vi "Save.vi"(6 "Force Single Line(T)":bool=TRUE, 7 "Channel Prefix(\"\")":string, 8 "error in (no error)":errorcluster, 9 "Group Prefix (\"\")":string, 10 "TDMS in":refnum<k34>, 11 "Data to Save":refnum<class "Data.lvclass">) -> (0 "error out":errorcluster, 2 "TDMS Out":refnum<k34>)   [LabVIEW 2020, in "TDMS.lvlib"]
doc: "Save 'Data to Save' to 'TDMS in'."
uses:
  TDMS.lvlib
  PPL/HDH.Data.Generic.lvlibp/Data.lvclass
  PPL/HDH.Data.Generic.lvlibp/Generic Data/Generic Array Data/Generic Array Data.lvclass
  PPL/HDH.Data.Generic.lvlibp/Generic Data/Generic Data.lvclass
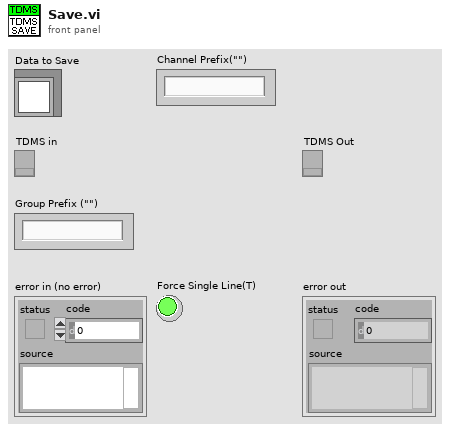
[diagram p1: front panel]
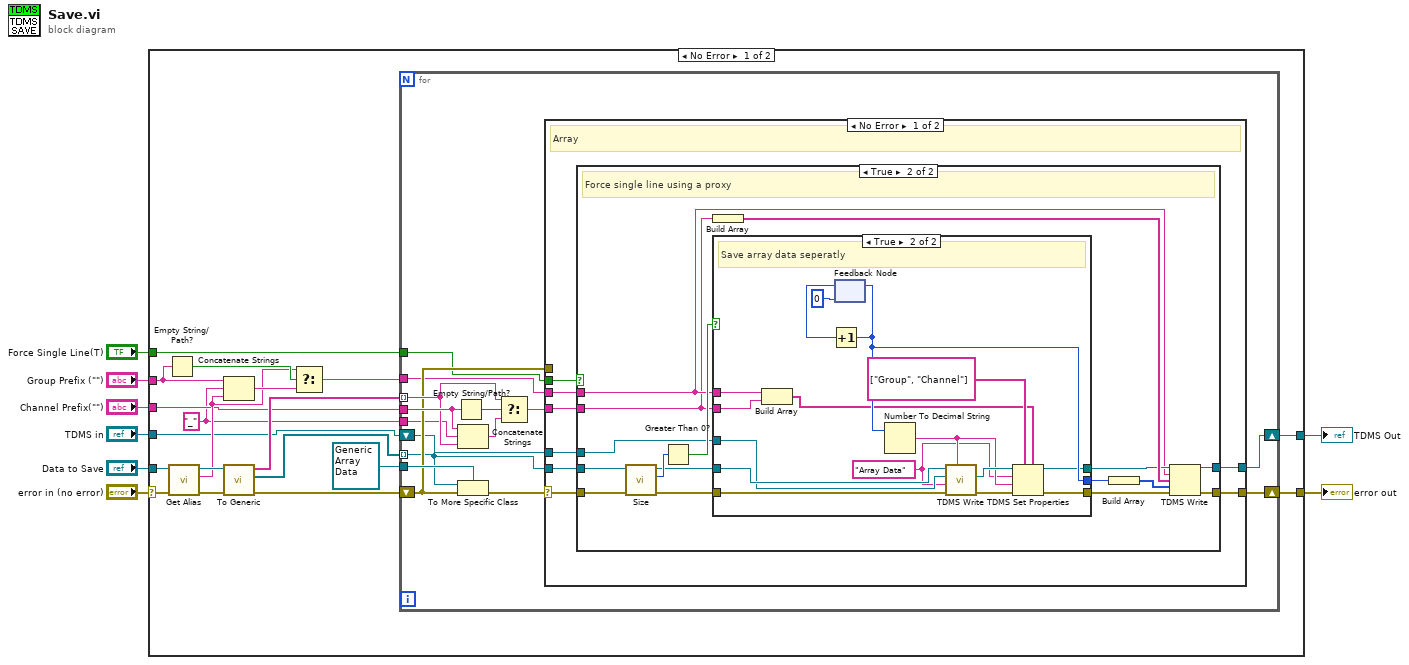
[diagram p0: block diagram]
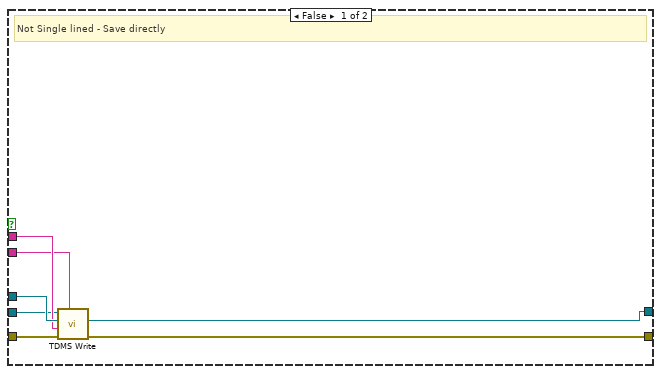
[diagram p2: hidden frame]
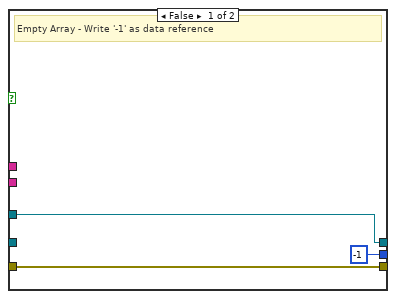
[diagram p3: hidden frame]
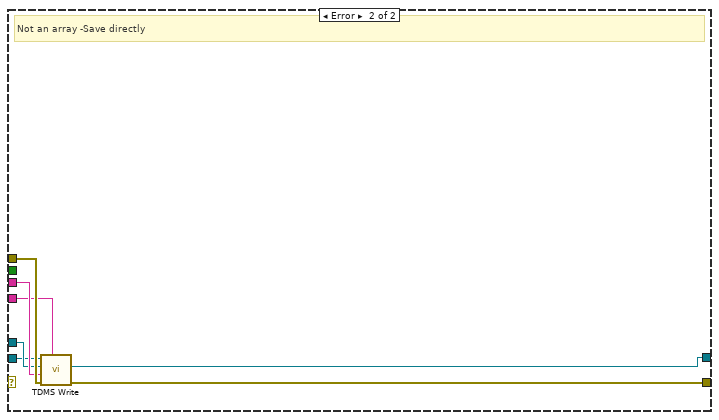
[diagram p4: hidden frame]
diagram:
  n1 = case shown="No Error" "error in (no error)" {
    selector: "error in (no error)" -> [w22 w101]
    tunnel: "Data to Save" -> [w27 _]
    tunnel: [w11 w101] -> w6
    tunnel: [w12 w100] -> w5
    tunnel: "TDMS in" -> [w13 w100]
    tunnel: "Group Prefix (\"\")" -> [w18 _]
    tunnel: "Channel Prefix(\"\")" -> [w14 _]
    tunnel: "Force Single Line(T)" -> [w10 _]
    frame No Error {
      w9 = "_" ("string")
      n2 = Empty String/Path?(string/path=w18) -> (empty?=w19:bool)
      n3 = call-dynamic "Get Alias.vi"("error in (no error)"=w22, "Data in"=w27) -> ("error out"=w21:errorcluster, "Alias"=w16:string, "Data out"=w26:refnum<class "Data.lvclass">)  [unwired: 7 in]
      n4 = Concatenate Strings(w18, w9, w16) -> (w17:string)
      n5 = call-dynamic "To Generic.vi"("error in (no error)"=w21, "Data in"=w26) -> ("error out"=w20:errorcluster, "Generic Data"=w25:refnum<class "Generic Data.lvclass">[], "Data Name"=w24:string[])  [unwired: 7 in]
      n6 = Select(t=w16, s=w19, f=w17) -> (s? t:f=w15:string)
      n7 = for {
        tunnel: w15 -> [w36]
        tunnel: w25 -> [w31] mode=indexing
        tunnel: w24 -> [w38] mode=indexing
        tunnel: refnum<class "Generic Array Data.lvclass"> refnum ("HDH.Data.Generic.lvlibp:Generic Array Data.lvclass") -> [w42]
        shift-right: [w32] -> w11
        shift-left: w20 -> [w37]
        tunnel: w14 -> [w39]
        shift-right: [w33] -> w12
        shift-left: w13 -> [w34]
        tunnel: w10 -> [w29]
        tunnel: w9 -> [w28]
        n8 = Empty String/Path?(string/path=w39) -> (empty?=w40:bool)
        n9 = Concatenate Strings(w39, w28, w38) -> (w41:string)
        n10 = To More Specific Class(target class=w42, reference=w31, error in=w37) -> (error out=w30:errorcluster)  [unwired: 1 out]
        n11 = Select(t=w38, s=w40, f=w41) -> (s? t:f=w35:string)
        n12 = case shown="No Error" w30 {
          selector: w30 -> [w49 _]
          tunnel: w37 -> [_ w99]
          tunnel: w36 -> [w46 w98]
          tunnel: w35 -> [w45 w97]
          tunnel: w34 -> [w48 w96]
          tunnel: [w47 w95] -> w33
          tunnel: [w43 w94] -> w32
          tunnel: w31 -> [w44 w93]
          tunnel: w29 -> [w50 _]
          frame No Error {
            # "Array"
            n13 = case shown="True" w50 {
              tunnel: w49 -> [w57 w70]
              tunnel: w48 -> [w56 w64]
              tunnel: [w55 w63] -> w47
              tunnel: w46 -> [w54 w59]
              tunnel: w45 -> [w53 w58]
              tunnel: w44 -> [w52 w73]
              tunnel: [w51 w62] -> w43
              frame False {
                # "Not Single lined - Save directly"
                n14 = call-dynamic "TDMS Write.vi"("Channel Name"=w53, "error in (no error)"=w57, "Group Name"=w54, "TDMS in"=w56, "Generic Data in"=w52) -> ("error out"=w51:errorcluster, "TDMS Out"=w55:refnum<k34>)  [unwired: 5 in]
              }
              frame True {
                # "Force single line using a proxy"
                n15 = call-dynamic "Size.vi"("error in (no error)"=w70, "Generic Data in"=w73) -> ("error out"=w61:errorcluster, "Size"=w72:i32, "Generic Data out"=w66:refnum<class "Generic Data.lvclass">)  [unwired: 7 in]
                n16 = Greater Than 0?(x=w72) -> (x > 0?=w71:bool)
                n17 = Build Array(w58) -> (w69:string[])
                n18 = case shown="True" w71 {
                  tunnel: [-1 w90] -> w68
                  tunnel: w66 -> [_ w89]
                  tunnel: [w75 w78] -> w65
                  tunnel: w64 -> [w75 w88]
                  tunnel: w61 -> [w74 w87]
                  tunnel: [w74 w77] -> w60
                  tunnel: w59 -> [_ w81]
                  tunnel: w58 -> [_ w80]
                  frame False {
                    # "Empty Array - Write '-1' as data reference"
                  }
                  frame True {
                    w83 = "Array Data" ("Group Name")
                    # "Save array data seperatly"
                    n19 = Build Array(w81, w80) -> (w79:string[])
                    n20 = feedback #1(0) -> (w91:i32)
                    n21 = Increment(x=w91) -> (x+1=w90:i32)
                    n22 = feedback-in #1(w90) -> ()
                    n23 = Number To Decimal String(number=w90) -> (decimal integer string=w84:string)  [unwired: 1 in]
                    n24 = call-dynamic "TDMS Write.vi"("Channel Name"=w84, "error in (no error)"=w87, "Group Name"=w83, "TDMS in"=w88, "Generic Data in"=w89) -> ("error out"=w86:errorcluster, "TDMS Out"=w85:refnum<k34>)  [unwired: 5 in]
                    n25 = TDMS Set Properties(5:w79, 7:string[] ["Group", "Channel"] ("property names"), 8:w86, 9:w84, 10:w83, 11:w85) -> (0:w77:errorcluster, 3:w78:refnum<k34>)  [unwired: 2 out]
                  }
                }
                n26 = Build Array(w68) -> (w67:i32[])
                n27 = TDMS Write(0:w65, 5:w59, 7:w69, 9:w67, 11:w60) -> (4:w63:refnum<k34>, 15:w62:errorcluster)  [unwired: 1 in, 2 out]
              }
            }
          }
          frame Error {
            # "Not an array -Save directly"
            n28 = call-dynamic "TDMS Write.vi"("Channel Name"=w97, "error in (no error)"=w99, "Group Name"=w98, "TDMS in"=w96, "Generic Data in"=w93) -> ("error out"=w94:errorcluster, "TDMS Out"=w95:refnum<k34>)  [unwired: 5 in]
          }
        }
      }
    }
    frame Error {
    }
  }
  "error out" <- w6
  "TDMS Out" <- w5
